vi "FindBlobs.vi"(10 "Vision Target":enum16{"Pegs", "Gears"}(ring), 11 "Image In":T2) -> (2 "Blob Data":T1, 3 "Image Out":T2)   [LabVIEW 2016]
uses:
  <vilib>/vision/Image Controls.llb/IMAQ Image.ctl
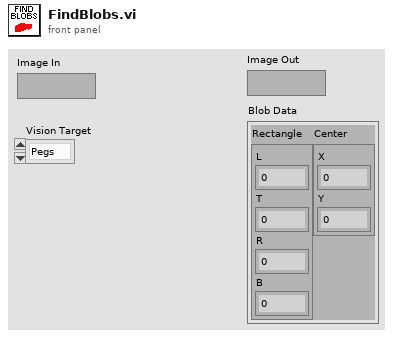
[diagram p1: front panel]
types:
  T1 = cluster{"Rectangle":cluster{"L":dbl, "T":dbl, "R":dbl, "B":dbl}, "Center":cluster{"X":dbl, "Y":dbl}}
  T2 = typedef "IMAQ Image.ctl" = refnum<image>
  T3 = typedef "Particle Parameters" = i32
  T4 = cluster{"Left":dbl, "Top":dbl, "Right":dbl, "Bottom":dbl}
  T5 = cluster{"Numeric":dbl, "Numeric":dbl, "Numeric":dbl, "Numeric":dbl}
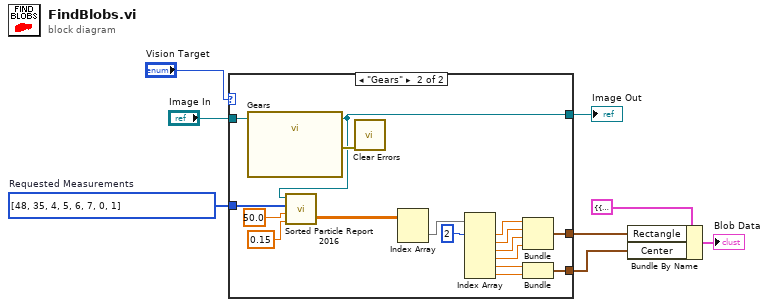
[diagram p0: block diagram]
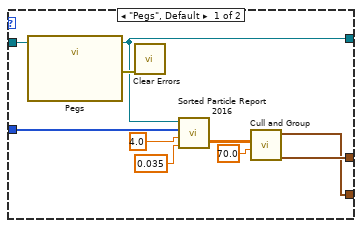
[diagram p2: hidden frame]
diagram:
  w6 = T3[] [48, 35, 4, 5, 6, 7, 0, 1] items=["Center of Mass X", "Center of Mass Y", "First Pixel X", "First Pixel Y", "Bounding Rect Left", "Bounding Rect Top", "Bounding Rect Right", "Bounding Rect Bottom", "Max Feret Diameter Start X", "Max Feret Diameter Start Y", "Max Feret Diameter End X", "Max Feret Diameter End Y", "Max Horiz. Segment Length Left", "Max Horiz. Segment Length Right", "Max Horiz. Segment Length Row", "-", "Bounding Rect Width", "Bounding Rect Height", "Bounding Rect Diagonal", "Perimeter", "Convex Hull Perimeter", "Holes' Perimeter", "Max Feret Diameter", "Equivalent Ellipse Major Axis", "Equivalent Ellipse Minor Axis", "Equivalent Ellipse Minor Axis (Feret)", "Equivalent Rect Long Side", "Equivalent Rect Short Side", "Equivalent Rect Diagonal", "Equivalent Rect Short Side (Feret)", "Average Horiz. Segment Length", "Average Vert. Segment Length", "Hydraulic Radius", "Waddel Disk Diameter", "-", "Area", "Holes' Area", "Particle & Holes' Area", "Convex Hull Area", "Image Area", "-", "Number of Holes", "Number of Horiz. Segments", "Number of Vert. Segments", "-", "Orientation", "Max Feret Diameter Orientation", "-", "% Area/Image Area", "% Area/(Particle & Holes' Area)", "Ratio of Equivalent Ellipse Axes", "Ratio of Equivalent Rect Sides", "-", "Elongation Factor", "Compactness Factor", "Heywood Circularity Factor", "Type Factor", "-", "Sum X", "Sum Y", "Sum XX", "Sum XY", "Sum YY", "Sum XXX", "Sum XXY", "Sum XYY", "Sum YYY", "-", "Moment of Inertia XX", "Moment of Inertia XY", "Moment of Inertia YY", "Moment of Inertia XXX", "Moment of Inertia XXY", "Moment of Inertia XYY", "Moment of Inertia YYY", "Norm. Moment of Inertia XX", "Norm. Moment of Inertia XY", "Norm. Moment of Inertia YY", "Norm. Moment of Inertia XXX", "Norm. Moment of Inertia XXY", "Norm. Moment of Inertia XYY", "Norm. Moment of Inertia YYY", "Hu Moment 1", "Hu Moment 2", "Hu Moment 3", "Hu Moment 4", "Hu Moment 5", "Hu Moment 6", "Hu Moment 7"]  # Requested Measurements
  n1 = case shown="\"Gears\"" "Vision Target" {
    tunnel: "Image In" -> [w17 w35]
    tunnel: w6 -> [w14 w33]
    tunnel: [w11 w19] -> w5
    tunnel: [w10 w21] -> w2
    tunnel: [w9 w20] -> w1
    frame "Pegs", Default {
      n2 = call "Pegs"("Image In"=w17) -> ("Image Out"=w11:T2, "error out"=w18:errorcluster)  [unwired: 25 in]
      n3 = call <vilib>:"Clear Errors.vi"("error in (no error)"=w18) -> ()  [unwired: 5 in, 2 out]
      n4 = call "Sorted Particle Report 2016.vi"("Min Area Size %"=0.035, "Particle Count Limit"=4.0, "Pixel Measurements"=w14, "Image in"=w11) -> ("Sorted Data"=w13:dbl[][])  [unwired: 1 out]
      n5 = call "Cull and Group.vi"("Score Cutoff"=70.0, "Sorted Data"=w13) -> ("Rect"=w10:T4, "Center"=w9:cluster{"X":dbl, "Y":dbl})  [unwired: 6 in, 2 out]
    }
    frame "Gears" {
      n6 = call "Gears"("Image In"=w35) -> ("Image Out"=w19:T2, "error out"=w34:errorcluster)  [unwired: 25 in]
      n7 = call "Sorted Particle Report 2016.vi"("Min Area Size %"=0.15, "Particle Count Limit"=50.0, "Pixel Measurements"=w33, "Image in"=w19) -> ("Sorted Data"=w30:dbl[][])  [unwired: 1 out]
      n8 = call <vilib>:"Clear Errors.vi"("error in (no error)"=w34) -> ()  [unwired: 5 in, 2 out]
      n9 = Index Array(array=w30) -> (element=w29:dbl[])  [unwired: 2 in]
      n10 = Index Array(array=w29, index #1=2 ("index")) -> (element #1=w27:dbl, element #2=w26:dbl, element #3=w25:dbl, element #4=w24:dbl, element #5=w23:dbl, element #6=w22:dbl)  [unwired: 5 in]
      n11 = Bundle("Numeric"=w27, "Numeric"=w26, "Numeric"=w25, "Numeric"=w24) -> (w21:T5)  [unwired: 1 in]
      n12 = Bundle("Numeric"=w23, "Numeric"=w22) -> (w20:cluster{"Numeric":dbl, "Numeric":dbl})  [unwired: 1 in]
    }
  }
  "Image Out" <- w5
  n13 = Bundle By Name(cluster=T1 {"Rectangle"={"L"=0.0, "T"=0.0, "R"=0.0, "B"=0.0}, "Center"={"X"=0.0, "Y"=0.0}} ("Blob Data"), "Rectangle"=w2, "Center"=w1) -> (→"Blob Data":T1)
